vi "Reset to Default Value.vi"(8 "错误输入（无错误）":errorcluster, 11 "Ctl Ref In":refnum<vi>) -> (0 "错误输出":errorcluster, 3 "Ctl Ref Out":refnum<vi>)   [LabVIEW 2012, in "CtrlRef.lvlib"]
uses:
  CtrlRef.lvlib
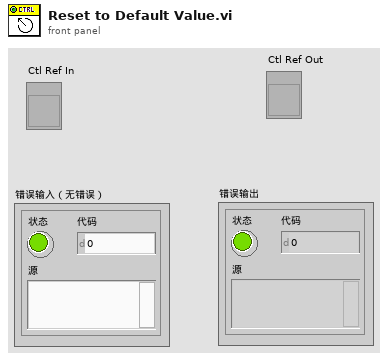
[diagram p1: front panel]
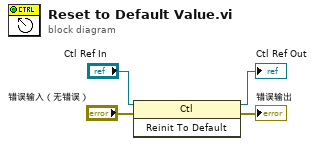
[diagram p0: block diagram]
diagram:
  n1 = invoke class="Ctl" method="Reinit To Default"(reference="Ctl Ref In", error in="错误输入（无错误）") -> (reference out=→"Ctl Ref Out":refnum<vi>, error out=→"错误输出":errorcluster)  [unwired: 1 in, 1 out]
